vi "BRig_dataLC_ENL_First_Delay_l1.vi"() -> (2 "output_ENL_First_Delay":i32)   [LabVIEW 2014]
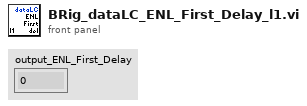
[diagram p1: front panel]
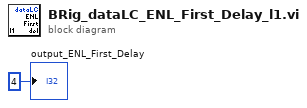
[diagram p0: block diagram]
diagram:
  "output_ENL_First_Delay" <- 4 ("output_iBlock")
